vi "testttt_Init.vi"(8 "ErrorIn":errorcluster caption="Error In", 11 "ObjectIn":refnum<class "testttt.lvclass"> caption="Object In") -> (0 "ErrorOut":errorcluster caption="Error Out", 3 "ObjectOut":refnum<class "testttt.lvclass"> caption="Object Out")   [LabVIEW 2018, in "testttt.lvclass"]
uses:
  testttt.lvclass
  testttt.lvclass/testttt.ctl
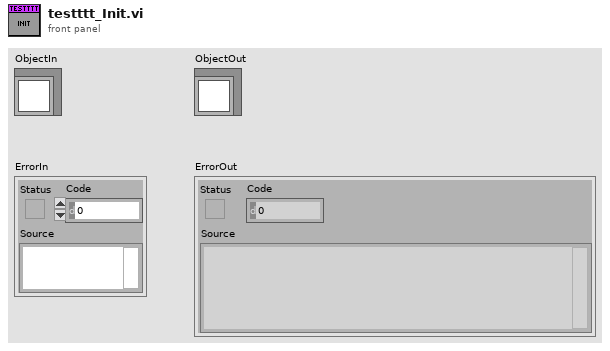
[diagram p1: front panel]
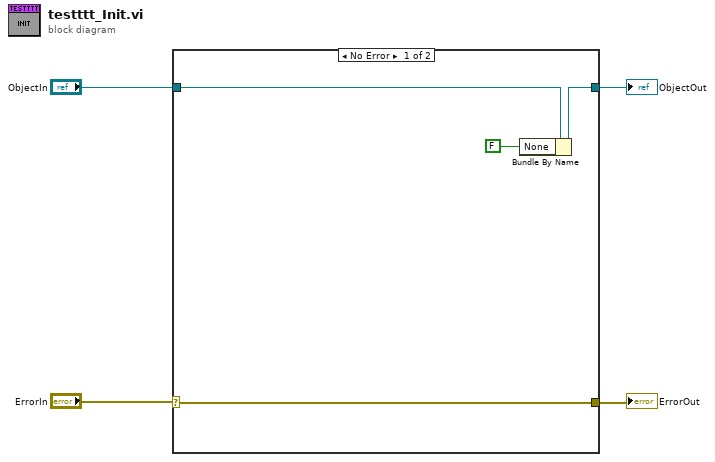
[diagram p0: block diagram]
diagram:
  n1 = case shown="No Error" "ErrorIn" {
    selector: "ErrorIn" -> [w8 w10]
    tunnel: "ObjectIn" -> [w5 w9]
    tunnel: [w7 w9] -> w1
    tunnel: [w8 w10] -> w3
    frame No Error {
      n2 = Bundle By Name(cluster=w5, "None"=FALSE) -> (w7:refnum<class "testttt.lvclass">)
    }
    frame Error {
    }
  }
  "ObjectOut" <- w1
  "ErrorOut" <- w3
